vi "Destructor.vi"(8 "error in":errorcluster, 11 "BooleanMeasureLimit":refnum<class "BooleanMeasureLimit.lvclass">) -> (0 "error out":errorcluster)   [LabVIEW 2021, in "ProligentXMLGenerator.lvlib" / "BooleanMeasureLimit.lvclass"]
uses:
  BooleanMeasureLimit.lvclass
  BooleanMeasureLimit.lvclass/BooleanMeasureLimit.ctl
  MeasureLimit/MeasureLimit.lvclass
  C:/Projects/proligent-xml-generator-labview/src/ProligentXMLGenerator/Measure/MeasureLimit/MeasureLimit.lvclass
  C:/Projects/proligent-xml-generator-labview/src/ProligentXMLGenerator/Measure/BooleanMeasureLimit/BooleanMeasureLimit.lvclass
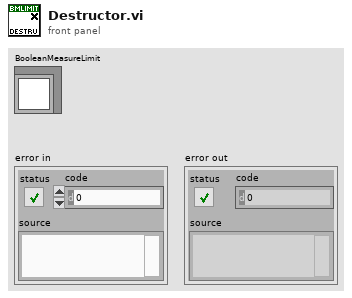
[diagram p1: front panel]
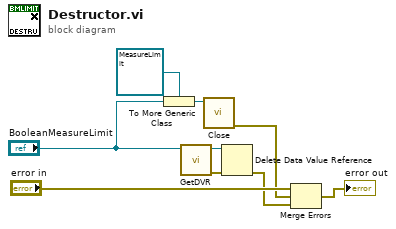
[diagram p0: block diagram]
diagram:
  n1 = To More Generic Class(target class=refnum<class "MeasureLimit.lvclass"> refnum ("ProligentResultProcessor:MeasureLimit"), reference="BooleanMeasureLimit") -> (generic class reference=w3:refnum<class "MeasureLimit.lvclass">)
  n2 = call "GetDVR.vi"("BooleanMeasureLimit"="BooleanMeasureLimit") -> ("error out"=w6:errorcluster, "DVRReference"=w7:refnum<data-value>)  [unwired: 9 in]
  n3 = call "Close.vi"("MeasureLimit"=w3) -> ("error out"=w5:errorcluster)  [unwired: 10 in]
  n4 = Delete Data Value Reference(data value reference=w7, error in=w6) -> (error out=w4:errorcluster)  [unwired: 1 out]
  n5 = Merge Errors("error in", w5, w4) -> (→"error out":errorcluster)
